vi "Create Arbitrary Waveform.vi"(6 "Timeout (10000 ms)":u32=10000, 8 "error in (no error)":errorcluster, 9 "Arbitrary Waveform Data":dbl[](array[numeric]), 10 "Arbitrary Waveform Name (\"ARB1\")":string="ARB1", 11 "VISA resource name":refnum<visa-resource-name>) -> (0 "error out":errorcluster, 3 "VISA resource name out":refnum<visa-resource-name>)   [LabVIEW 2017, in "Keithley 3390.lvlib"]
doc: "Creates and saves an arbitrary (user-defined) waveform in non-volatile memory. \n\n<B>Remarks:</B>\n \n(1) Data is scaled and normalized so that the waveform will be centered around y=0. Model 3390 has a 14-bit digitizer and will be scaled from -8191 to + 8191.\n\n(2) Call Configure Arbitrary Waveform VI to set the arbitrary waveform as the active function.\n\n(3) Creates an arbitrary waveform in non-volatile memory and because of this, the waveform will remain stored on the instrument until deleted. If any sensitive information is contained in the arbitrary waveform, it is recommended that the waveform be deleted when finished"
uses:
  Keithley 3390.lvlib
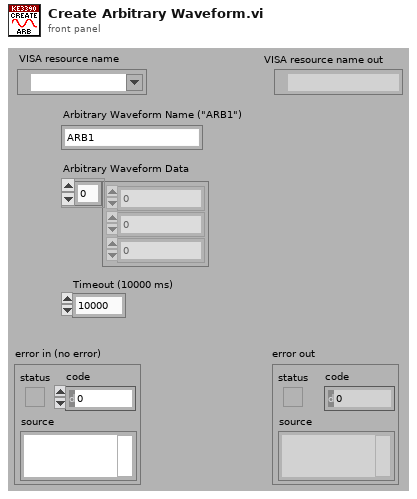
[diagram p1: front panel]
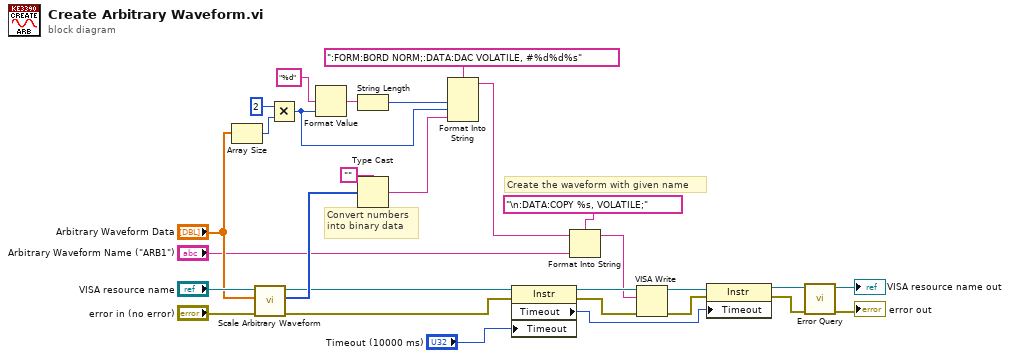
[diagram p0: block diagram]
diagram:
  # "Convert numbers\ninto binary data"
  # "Create the waveform with given name"
  n1 = Array Size(array="Arbitrary Waveform Data") -> (size(s)=w28:i32)
  n2 = call "Scale Arbitrary Waveform.vi"("error in (no error)"="error in (no error)", "Arbitrary Waveform Data"="Arbitrary Waveform Data", "VISA resource name"="VISA resource name") -> ("error out"=w20:errorcluster, "Scaled Arbitrary Waveform Data"=w22:i16[], "VISA resource name out"=w21:refnum<visa-resource-name>)  [unwired: 6 in]
  n3 = Multiply(x=2, y=w28) -> (x*y=w11:i32)
  n4 = Format Value(format string="%d", value (0)=w11) -> (output string=w25:string)  [unwired: 1 in]
  n5 = String Length(string=w25) -> (length=w12:i32)
  n6 = Type Cast(type="", x=w22) -> (*(type *) &x=w10:string)
  n7 = Format Into String(format string=":FORM:BORD NORM;:DATA:DAC VOLATILE, #%d%d%s" ("string"), w12, w11, w10) -> (resulting string=w8:string)  [unwired: 2 in, 1 out]
  n8 = property class="Instr"(reference=w21, error in=w20, "Timeout"="Timeout (10000 ms)") -> (reference out=w18:refnum<visa-resource-name>, error out=w19:errorcluster, "Timeout"=w15:u32)
  n9 = Format Into String(format string="\n:DATA:COPY %s, VOLATILE;", initial string=w8, "Arbitrary Waveform Name (\"ARB1\")") -> (resulting string=w6:string)  [unwired: 1 in, 1 out]
  n10 = VISA Write(VISA resource name=w18, write buffer=w6, error in (no error)=w19) -> (VISA resource name out=w17:refnum<visa-resource-name>, error out=w16:errorcluster)  [unwired: 1 out]
  n11 = property class="Instr"(reference=w17, error in=w16, "Timeout"=w15) -> (reference out=w4:refnum<visa-resource-name>, error out=w3:errorcluster)
  n12 = call "Error Query.vi"("error in (no error)"=w3, "VISA resource name"=w4) -> ("error out"=→"error out":errorcluster, "VISA resource name out"=→"VISA resource name out":refnum<visa-resource-name>)  [unwired: 6 in, 2 out]
